vi "Configuration File Path Parameter Check.vi"(0 "Parameter Name":string, 1 "Component Root Path":path, 5 "Specified Path in Configuration File":path, 7 "Configuration File Path":path, 11 "error in (no error)":errorcluster) -> (6 "dup Specified Path in Configuration File":path, 8 "dup Configuration File Path":path, 15 "error out":errorcluster)   [LabVIEW 2017, in "CL_G3_VIComponentBuilder.lvlib"]
uses:
  CL_G3_VIComponentBuilder.lvlib
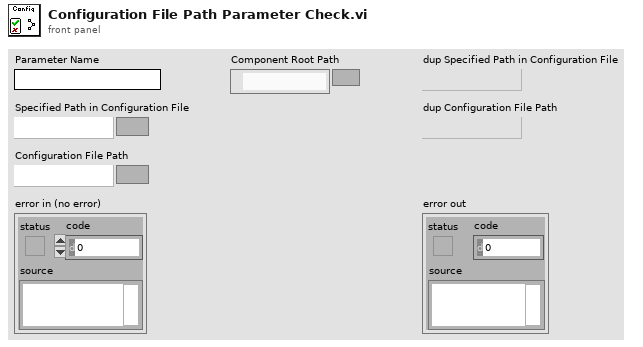
[diagram p1: front panel]
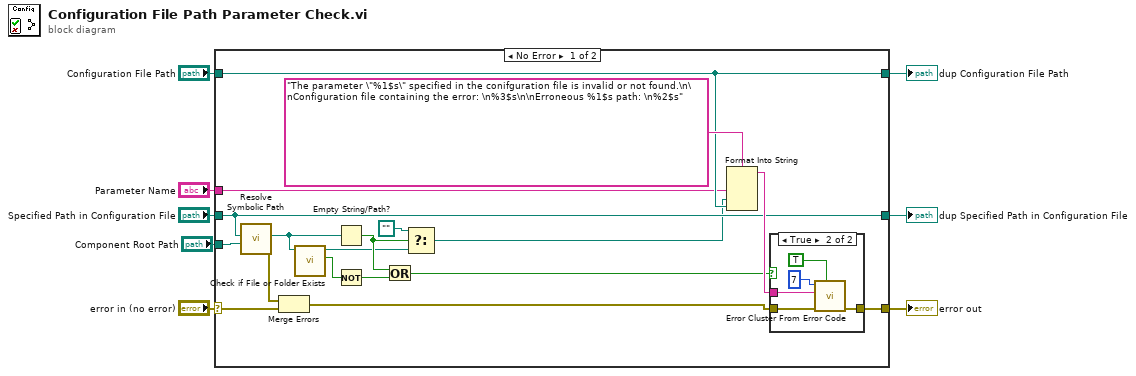
[diagram p0: block diagram]
diagram:
  n1 = case shown="No Error" "error in (no error)" {
    selector: "error in (no error)" -> [w12 w35]
    tunnel: [w24 w35] -> w7
    tunnel: "Configuration File Path" -> [w19 w34]
    tunnel: "Parameter Name" -> [w16 _]
    tunnel: "Specified Path in Configuration File" -> [w20 w33]
    tunnel: [w20 w33] -> w3
    tunnel: [w19 w34] -> w2
    tunnel: "Component Root Path" -> [w9 _]
    frame No Error {
      n2 = call "Resolve Symbolic Path.vi"("Component Root Path"=w9, "Path In"=w20) -> ("error out"=w11:errorcluster, "Path Out"=w22:path)  [unwired: 8 in]
      n3 = Merge Errors(w11, w12) -> (w10:errorcluster)
      n4 = call <vilib>:"Check if File or Folder Exists.vi"("path"=w22) -> ("file or folder exists?"=w23:bool, "dup path"=w14:path)  [unwired: 8 in, 1 out]
      n5 = Empty String/Path?(string/path=w22) -> (empty?=w17:bool)
      n6 = Not(x=w23) -> (.not. x?=w18:bool)
      n7 = Or(x=w17, y=w18) -> (x .or. y?=w21:bool)
      n8 = Select(t=path "", s=w17, f=w14) -> (s? t:f=w13:path)
      n9 = Format Into String(format string="The parameter \"%1$s\" specified in the conifguration file is invalid or not found.\n\nConfiguration file containing the error: \n%3$s\n\nErroneous %1$s path: \n%2$s", w16, w13, w19) -> (resulting string=w26:string)  [unwired: 2 in, 1 out]
      n10 = case shown="True" w21 {
        tunnel: w26 -> [_ w31]
        tunnel: w10 -> [w27 w29]
        tunnel: [w27 w28] -> w24
        frame False {
        }
        frame True {
          n11 = call <vilib>:"Error Cluster From Error Code.vi"("show call chain? (False)"=TRUE, "error in (no error)"=w29, "error message (\"\")"=w31, "error code (0)"=7) -> ("error out"=w28:errorcluster)  [unwired: 5 in]
        }
      }
    }
    frame Error {
    }
  }
  "error out" <- w7
  "dup Specified Path in Configuration File" <- w3
  "dup Configuration File Path" <- w2
